vi "CLC_JIO_Recode_ALL_addSG.vi"(0 "UD_att":i32=255, 1 "pol":u16, 2 "Mode":enum16{"Standy", "Tx", "Rx"}(ring)=enum."Tx", 3 "Function":T1, 5 "com_att":i32=255, 7 "ele_att":i32=255, 9 "SG Power":i32=-10, 11 "error in":errorcluster, 13 "Enable?":bool, 14 "FileName":string="SingleCh_") -> (15 "error out":errorcluster)   [LabVIEW 2023, in "CLC_JIO_FTDI.lvlib"]
uses:
  CLC_JIO_FTDI.lvlib
  CTL/JIO_FPGA_FTDI.ctl
panel:
  out "standard error":string
  out "floder?":bool
  out "standard output":string
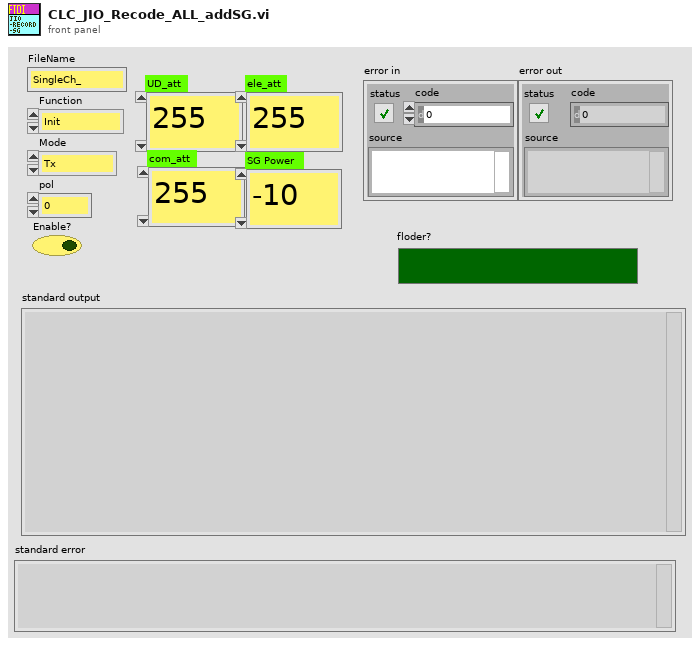
[diagram p1: front panel]
types:
  T1 = typedef "JIO_FPGA_FTDI.ctl" = enum16{"Init", "Close", "UD", "BFIC"}
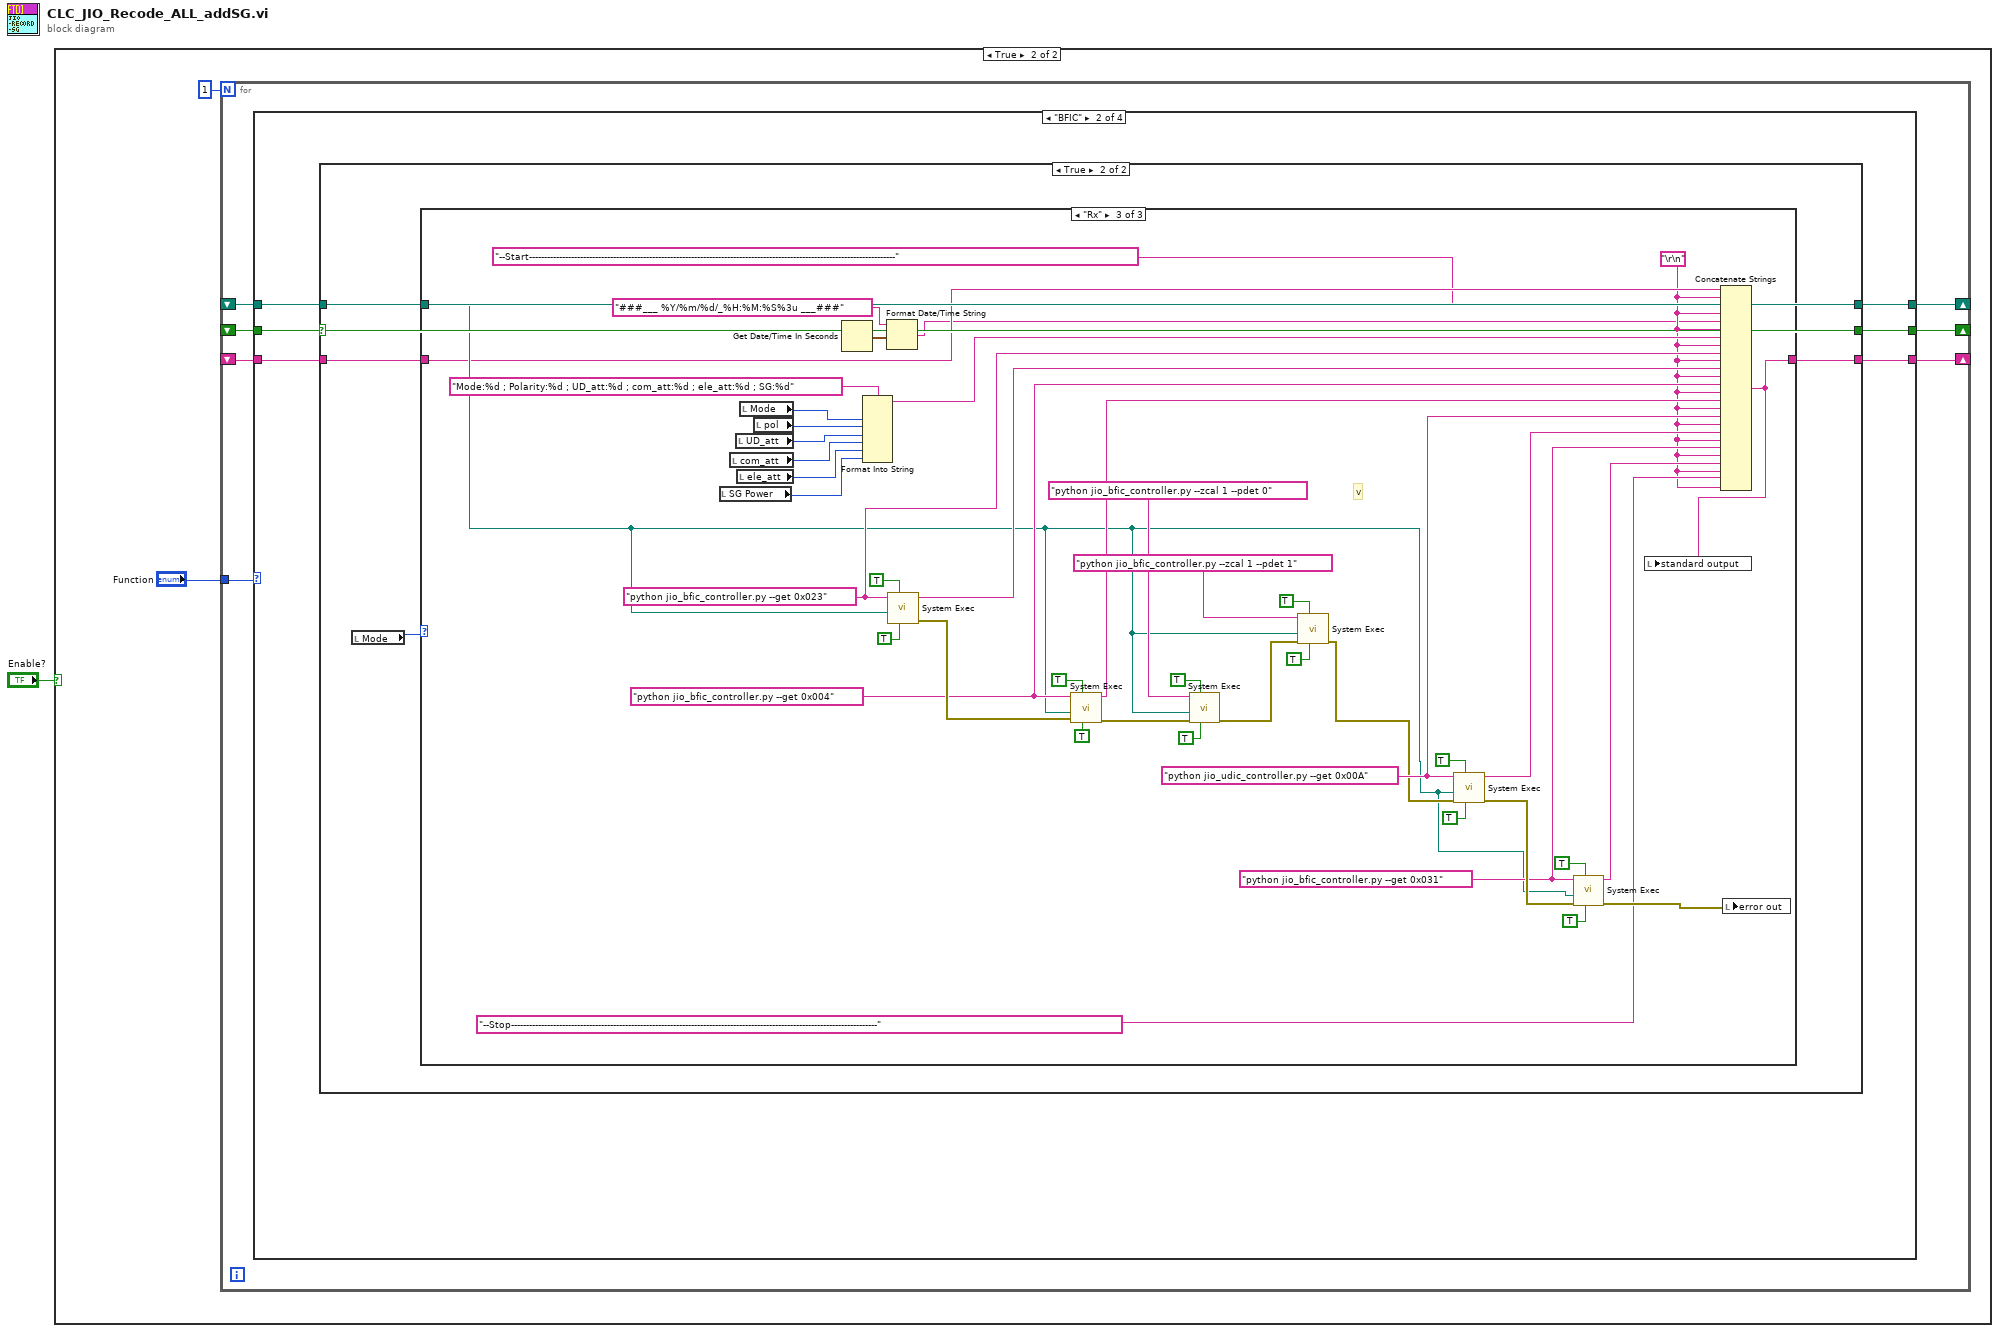
[diagram p0: block diagram]
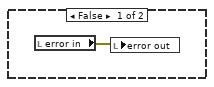
[diagram p2: hidden frame]
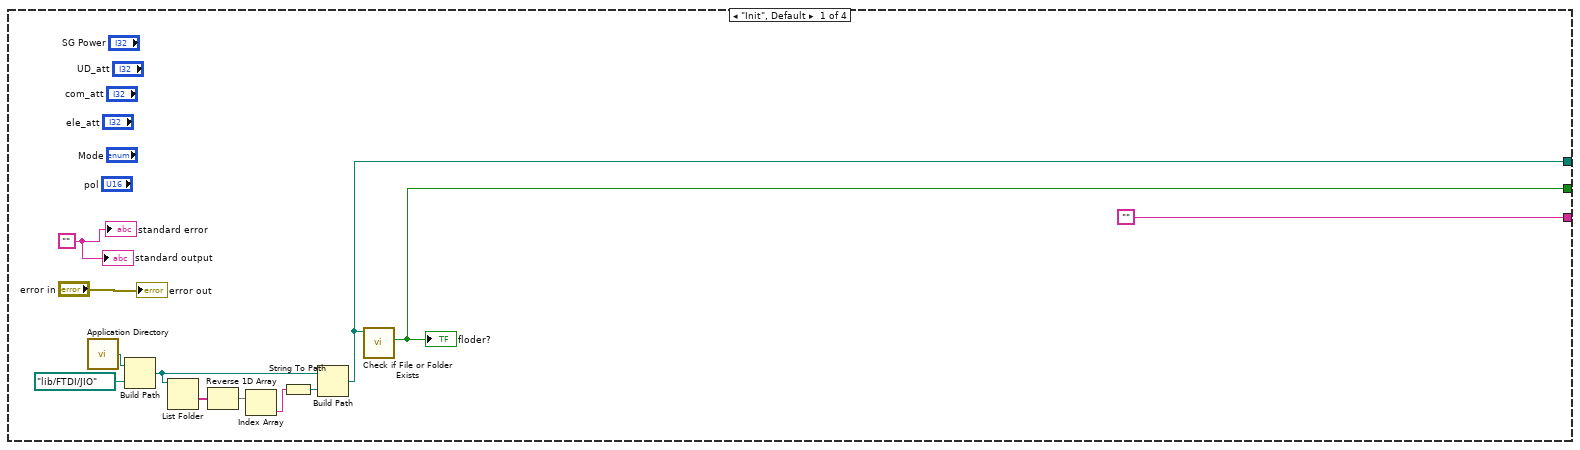
[diagram p3: hidden frame]
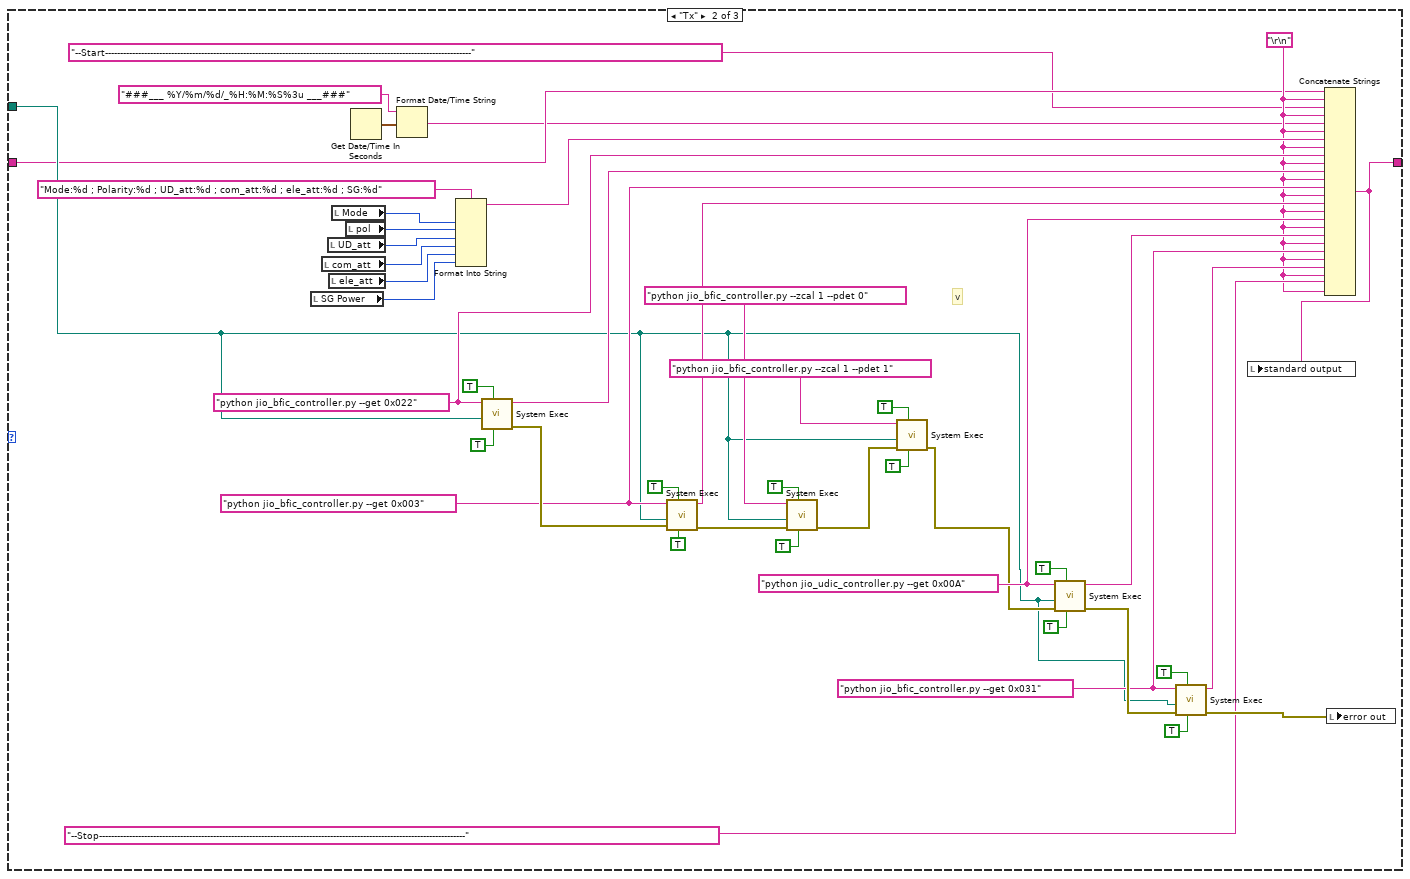
[diagram p6: hidden frame]
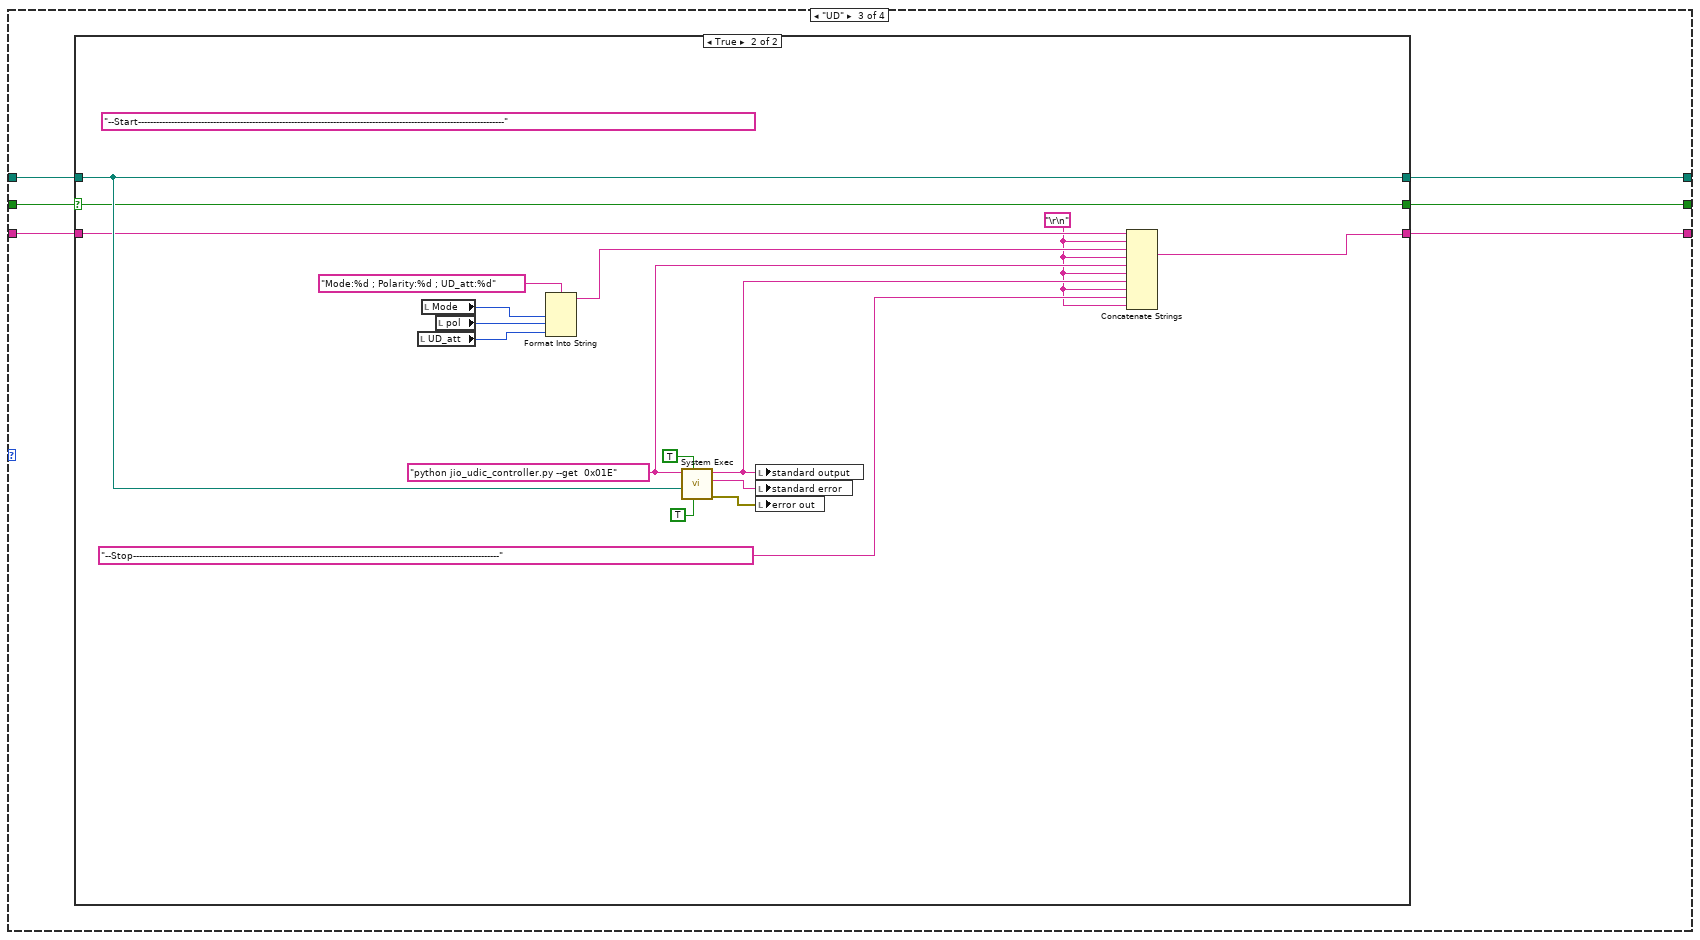
[diagram p7: hidden frame]
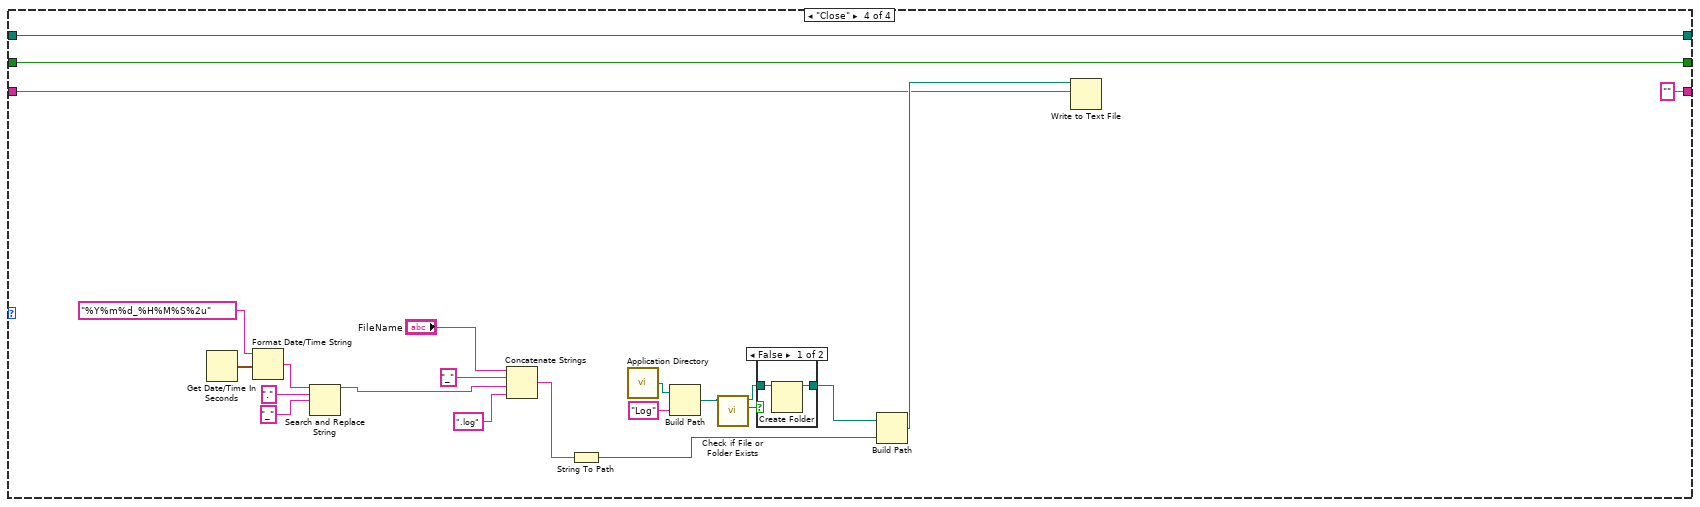
[diagram p9: hidden frame]
diagram:
  n1 = case shown="True" "Enable?" {
    frame False {
      n2 = local read "error in"() -> (w2:errorcluster)
      n3 = local write "error out"(w2) -> ()
    }
    frame True {
      n4 = for {
        N: 1 -> [_]
        tunnel: "Function" -> [w11]
        shift-right: [w10] -> _
        shift-left: _ -> [w6]
        shift-right: [w9] -> _
        shift-left: _ -> [w7]
        shift-right: [w8] -> _
        shift-left: _ -> [w5]
        n5 = case shown="\"BFIC\"" w11 {
          tunnel: [w16 w27 w132 w155] -> w10
          tunnel: [w15 w26 w131 w156] -> w9
          tunnel: ["" w25 w130 ""] -> w8
          tunnel: w7 -> [_ w29 w134 w156]
          tunnel: w6 -> [_ w28 w133 w155]
          tunnel: w5 -> [_ w24 w129 w158]
          frame "Init", Default {
            w12 = ""
            n6 = call <vilib>:"Application Directory.vi"() -> ("Application Directory"=w22:path)
            n7 = Build Path(base path=w22, name or relative path=path "lib/FTDI/JIO") -> (appended path=w23:path)
            n8 = List Folder(path=w23) -> (folder names=w18:string[])  [unwired: 3 in, 3 out]
            n9 = Reverse 1D Array(array=w18) -> (reversed array=w19:string[])
            n10 = Index Array(array=w19) -> (element=w20:string)  [unwired: 1 in]
            n11 = String To Path(string=w20) -> (path=w21:path)
            n12 = Build Path(base path=w23, name or relative path=w21) -> (appended path=w16:path)
            n13 = call <vilib>:"Check if File or Folder Exists.vi"("path"=w16) -> ("file or folder exists?"=w15:bool)  [unwired: 8 in, 2 out]
            "floder?" <- w15
            "standard output" <- w12
            "error out" <- "error in"
            "standard error" <- w12
          }
          frame "BFIC" {
            n14 = case shown="True" w29 {
              selector: w29 -> [w31 w36]
              tunnel: w28 -> [w32 w37]
              tunnel: [w32 w37] -> w27
              tunnel: [w31 w36] -> w26
              tunnel: [w30 w34] -> w25
              tunnel: w24 -> [w30 w35]
              frame False {
              }
              frame True {
                n15 = local read "Mode"() -> (w33:enum16{"Standy", "Tx", "Rx"})
                n16 = case shown="\"Rx\"" w33 {
                  tunnel: w37 -> [_ w46 w91]
                  tunnel: w35 -> [w38 w41 w87]
                  tunnel: [w38 w56 w101] -> w34
                  frame "Standy", Default {
                  }
                  frame "Tx" {
                    w61 = "python jio_udic_controller.py --get 0x00A" ("string")
                    w59 = "python jio_bfic_controller.py --get 0x031" ("string")
                    w42 = "\r\n"
                    w70 = "python jio_bfic_controller.py --get 0x003" ("string")
                    w73 = "python jio_bfic_controller.py --get 0x022" ("string")
                    # "v"
                    n17 = local read "SG Power"() -> (w45:i32)
                    n18 = local read "com_att"() -> (w76:i32)
                    n19 = local read "UD_att"() -> (w79:i32)
                    n20 = local read "ele_att"() -> (w75:i32)
                    n21 = local read "Mode"() -> (w81:enum16{"Standy", "Tx", "Rx"})
                    n22 = local read "pol"() -> (w80:u16)
                    n23 = Get Date/Time In Seconds() -> (seconds since 1Jan1904=w44:timestamp)
                    n24 = Format Date/Time String(time format string (%c)="###___ %Y/%m/%d/_%H:%M:%S%3u ___###", seconds (now)=w44) -> (date/time string=w39:string)  [unwired: 1 in]
                    n25 = Format Into String(format string="Mode:%d ; Polarity:%d ; UD_att:%d ; com_att:%d ; ele_att:%d ; SG:%d" ("string"), w81, w80, w79, w76, w75, w45) -> (resulting string=w71:string)  [unwired: 2 in, 1 out]
                    n26 = call <vilib>:"System Exec.vi"("run minimized? (F)"=TRUE, "wait until completion? (T)"=TRUE, "working directory"=w46, "command line"=w73) -> ("error out"=w74:errorcluster, "standard output"=w69:string)  [unwired: 4 in, 2 out]
                    n27 = call <vilib>:"System Exec.vi"("run minimized? (F)"=TRUE, "wait until completion? (T)"=TRUE, "error in (no error)"=w74, "working directory"=w46, "command line"=w70) -> ("error out"=w51:errorcluster, "standard output"=w68:string)  [unwired: 3 in, 2 out]
                    n28 = call <vilib>:"System Exec.vi"("run minimized? (F)"=TRUE, "wait until completion? (T)"=TRUE, "error in (no error)"=w51, "working directory"=w46, "command line"="python jio_bfic_controller.py --zcal 1 --pdet 0" ("string")) -> ("error out"=w49:errorcluster)  [unwired: 3 in, 3 out]
                    n29 = call <vilib>:"System Exec.vi"("run minimized? (F)"=TRUE, "wait until completion? (T)"=TRUE, "error in (no error)"=w49, "working directory"=w46, "command line"="python jio_bfic_controller.py --zcal 1 --pdet 1" ("string")) -> ("error out"=w50:errorcluster)  [unwired: 3 in, 3 out]
                    n30 = call <vilib>:"System Exec.vi"("run minimized? (F)"=TRUE, "wait until completion? (T)"=TRUE, "error in (no error)"=w50, "working directory"=w46, "command line"=w61) -> ("error out"=w63:errorcluster, "standard output"=w60:string)  [unwired: 3 in, 2 out]
                    n31 = call <vilib>:"System Exec.vi"("run minimized? (F)"=TRUE, "wait until completion? (T)"=TRUE, "error in (no error)"=w63, "working directory"=w46, "command line"=w59) -> ("error out"=w62:errorcluster, "standard output"=w57:string)  [unwired: 3 in, 2 out]
                    n32 = Concatenate Strings(w41, w42, "--Start--------------------------------------------------------------------------------------------------------------------------" ("string"), w42, w39, w42, w71, w42, w73, w42, w69, w42, w70, w42, w68, w42, w61, w42, w60, w42, w59, w42, w57, w42, "--Stop--------------------------------------------------------------------------------------------------------------------------" ("string"), w42) -> (w56:string)
                    n33 = local write "standard output"(w56) -> ()
                    n34 = local write "error out"(w62) -> ()
                  }
                  frame "Rx" {
                    w106 = "python jio_udic_controller.py --get 0x00A" ("string")
                    w104 = "python jio_bfic_controller.py --get 0x031" ("string")
                    w86 = "\r\n"
                    w115 = "python jio_bfic_controller.py --get 0x004" ("string")
                    w118 = "python jio_bfic_controller.py --get 0x023" ("string")
                    # "v"
                    n35 = local read "SG Power"() -> (w90:i32)
                    n36 = local read "com_att"() -> (w121:i32)
                    n37 = local read "UD_att"() -> (w124:i32)
                    n38 = local read "ele_att"() -> (w120:i32)
                    n39 = local read "Mode"() -> (w126:enum16{"Standy", "Tx", "Rx"})
                    n40 = local read "pol"() -> (w125:u16)
                    n41 = Get Date/Time In Seconds() -> (seconds since 1Jan1904=w89:timestamp)
                    n42 = Format Into String(format string="Mode:%d ; Polarity:%d ; UD_att:%d ; com_att:%d ; ele_att:%d ; SG:%d" ("string"), w126, w125, w124, w121, w120, w90) -> (resulting string=w116:string)  [unwired: 2 in, 1 out]
                    n43 = Format Date/Time String(time format string (%c)="###___ %Y/%m/%d/_%H:%M:%S%3u ___###", seconds (now)=w89) -> (date/time string=w84:string)  [unwired: 1 in]
                    n44 = call <vilib>:"System Exec.vi"("run minimized? (F)"=TRUE, "wait until completion? (T)"=TRUE, "working directory"=w91, "command line"=w118) -> ("error out"=w119:errorcluster, "standard output"=w114:string)  [unwired: 4 in, 2 out]
                    n45 = call <vilib>:"System Exec.vi"("run minimized? (F)"=TRUE, "wait until completion? (T)"=TRUE, "error in (no error)"=w119, "working directory"=w91, "command line"=w115) -> ("error out"=w96:errorcluster, "standard output"=w113:string)  [unwired: 3 in, 2 out]
                    n46 = call <vilib>:"System Exec.vi"("run minimized? (F)"=TRUE, "wait until completion? (T)"=TRUE, "error in (no error)"=w96, "working directory"=w91, "command line"="python jio_bfic_controller.py --zcal 1 --pdet 0" ("string")) -> ("error out"=w94:errorcluster)  [unwired: 3 in, 3 out]
                    n47 = call <vilib>:"System Exec.vi"("run minimized? (F)"=TRUE, "wait until completion? (T)"=TRUE, "error in (no error)"=w94, "working directory"=w91, "command line"="python jio_bfic_controller.py --zcal 1 --pdet 1" ("string")) -> ("error out"=w95:errorcluster)  [unwired: 3 in, 3 out]
                    n48 = call <vilib>:"System Exec.vi"("run minimized? (F)"=TRUE, "wait until completion? (T)"=TRUE, "error in (no error)"=w95, "working directory"=w91, "command line"=w106) -> ("error out"=w108:errorcluster, "standard output"=w105:string)  [unwired: 3 in, 2 out]
                    n49 = call <vilib>:"System Exec.vi"("run minimized? (F)"=TRUE, "wait until completion? (T)"=TRUE, "error in (no error)"=w108, "working directory"=w91, "command line"=w104) -> ("error out"=w107:errorcluster, "standard output"=w102:string)  [unwired: 3 in, 2 out]
                    n50 = Concatenate Strings(w87, w86, "--Start--------------------------------------------------------------------------------------------------------------------------" ("string"), w86, w84, w86, w116, w86, w118, w86, w114, w86, w115, w86, w113, w86, w106, w86, w105, w86, w104, w86, w102, w86, "--Stop--------------------------------------------------------------------------------------------------------------------------" ("string"), w86) -> (w101:string)
                    n51 = local write "standard output"(w101) -> ()
                    n52 = local write "error out"(w107) -> ()
                  }
                }
              }
            }
          }
          frame "UD" {
            n53 = case shown="True" w134 {
              selector: w134 -> [w136 w149]
              tunnel: w133 -> [w137 w150]
              tunnel: [w137 w150] -> w132
              tunnel: [w136 w149] -> w131
              tunnel: [w135 w146] -> w130
              tunnel: w129 -> [w135 w148]
              frame False {
              }
              frame True {
                w138 = "\r\n"
                (unwired) "--Start--------------------------------------------------------------------------------------------------------------------------" ("string")
                w141 = "python jio_udic_controller.py --get  0x01E" ("string")
                n54 = local read "UD_att"() -> (w143:i32)
                n55 = local read "Mode"() -> (w145:enum16{"Standy", "Tx", "Rx"})
                n56 = local read "pol"() -> (w144:u16)
                n57 = Format Into String(format string="Mode:%d ; Polarity:%d ; UD_att:%d" ("string"), w145, w144, w143) -> (resulting string=w142:string)  [unwired: 2 in, 1 out]
                n58 = call <vilib>:"System Exec.vi"("run minimized? (F)"=TRUE, "wait until completion? (T)"=TRUE, "working directory"=w150, "command line"=w141) -> ("error out"=w151:errorcluster, "standard error"=w152:string, "standard output"=w140:string)  [unwired: 4 in, 1 out]
                n59 = local write "standard output"(w140) -> ()
                n60 = local write "standard error"(w152) -> ()
                n61 = local write "error out"(w151) -> ()
                n62 = Concatenate Strings(w148, w138, w142, w138, w141, w138, w140, w138, "--Stop--------------------------------------------------------------------------------------------------------------------------" ("string"), w138) -> (w146:string)
              }
            }
          }
          frame "Close" {
            n63 = Get Date/Time In Seconds() -> (seconds since 1Jan1904=w171:timestamp)
            n64 = Format Date/Time String(time format string (%c)="%Y%m%d_%H%M%S%2u", seconds (now)=w171) -> (date/time string=w169:string)  [unwired: 1 in]
            n65 = Search and Replace String(input string=w169, search string=".", replace string="_") -> (result string=w166:string)  [unwired: 5 in, 3 out]
            n66 = Concatenate Strings("FileName", "_" ("delimiter (\\t)"), w166, ".log" ("delimiter (\\t)")) -> (w174:string)
            n67 = String To Path(string=w174) -> (path=w175:path)
            n68 = call <vilib>:"Application Directory.vi"() -> ("Application Directory"=w173:path)
            n69 = Build Path(base path=w173, name or relative path="Log") -> (appended path=w163:path)
            n70 = call <vilib>:"Check if File or Folder Exists.vi"("path"=w163) -> ("file or folder exists?"=w165:bool, "dup path"=w164:path)  [unwired: 8 in, 1 out]
            n71 = case shown="False" w165 {
              tunnel: w164 -> [w178 w179]
              tunnel: [w177 w179] -> w162
              frame False {
                n72 = Create Folder(path (use dialog)=w178) -> (created path=w177:path)  [unwired: 2 in, 2 out]
              }
              frame True {
              }
            }
            n73 = Build Path(base path=w162, name or relative path=w175) -> (appended path=w161:path)
            n74 = Write to Text File(file (use dialog)=w161, text=w158) -> ()  [unwired: 2 in, 3 out]
          }
        }
      }
    }
  }
